vi "(Sub) Write CMD.vi"(7 "State":T1, 8 "error in (no error)":errorcluster caption="에러 입력(에러 없음)", 10 "Write Data":string) -> (0 "error out":errorcluster caption="에러 출력", 1 "Read Byte":i32, 2 "CMD":string, 3 "Write CMD":string)   [LabVIEW 2017]
uses:
  Controls/(Ctrl) State_Write CMD.ctl
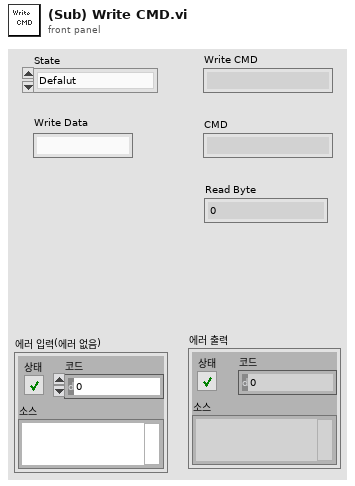
[diagram p1: front panel]
types:
  T1 = typedef "(Ctrl) State_Write CMD.ctl" = enum16{"Defalut", "Set KV", "Set mA", "Get KV", "Get mA", "Get ADC", "HV On", "HV Off", "System State", "HV State", "Opration Mode"}
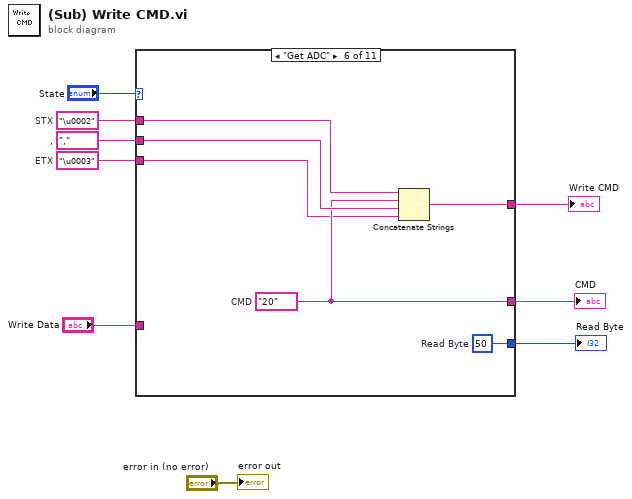
[diagram p0: block diagram]
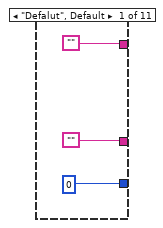
[diagram p2: hidden frame]
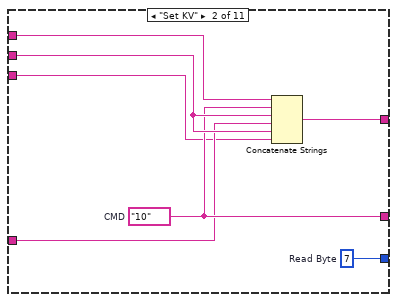
[diagram p3: hidden frame]
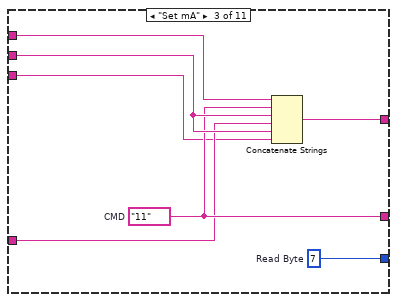
[diagram p4: hidden frame]
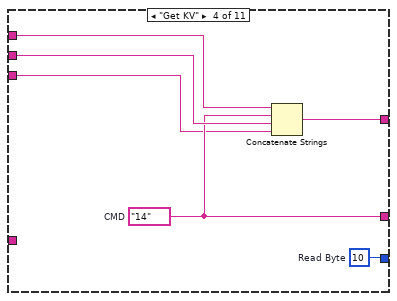
[diagram p5: hidden frame]
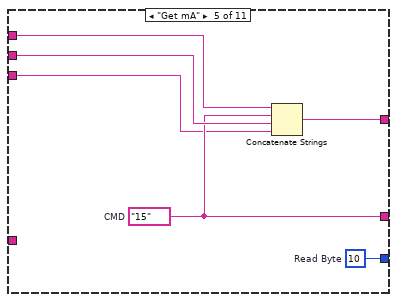
[diagram p6: hidden frame]
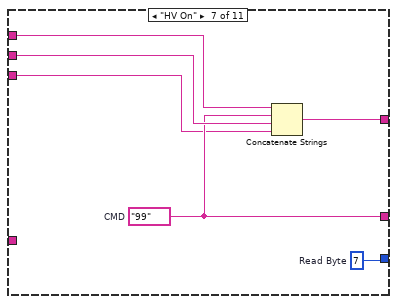
[diagram p7: hidden frame]
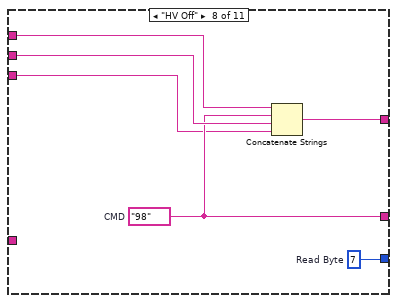
[diagram p8: hidden frame]
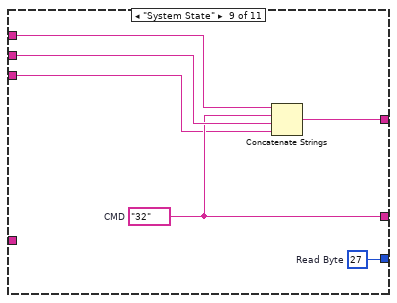
[diagram p9: hidden frame]
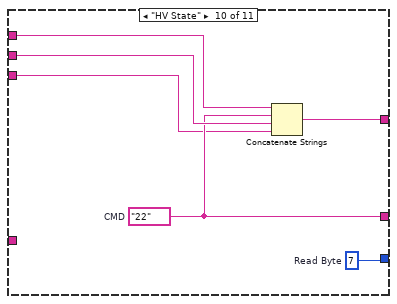
[diagram p10: hidden frame]
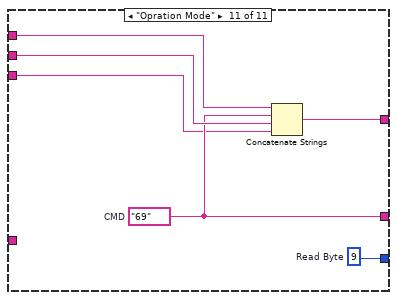
[diagram p11: hidden frame]
diagram:
  w6 = ","  # ,
  w1 = "\u0003"  # ETX
  w7 = "\u0002"  # STX
  n1 = case shown="\"Get ADC\"" "State" {
    tunnel: w7 -> [_ w18 w25 w31 w37 w43 w49 w55 w61 w67 w73]
    tunnel: w6 -> [_ w19 w26 w32 w38 w44 w50 w56 w62 w68 w74]
    tunnel: ["" w17 w24 w30 w36 w42 w48 w54 w60 w66 w72] -> w5
    tunnel: ["" w16 w23 w29 w35 w41 w47 w53 w59 w65 w71] -> w4
    tunnel: "Write Data" -> [_ w15 w22 _ _ _ _ _ _ _ _]
    tunnel: [0 w14 w21 w28 w34 w40 w46 w52 w58 w64 w70] -> w2
    tunnel: w1 -> [_ w13 w20 w27 w33 w39 w45 w51 w57 w63 w69]
    frame "Defalut", Default {
    }
    frame "Set KV" {
      w14 = 7  # Read Byte
      w16 = "10"  # CMD
      n2 = Concatenate Strings(w18, w16, w19, w15, w19, w13) -> (w17:string)
    }
    frame "Set mA" {
      w21 = 7  # Read Byte
      w23 = "11"  # CMD
      n3 = Concatenate Strings(w25, w23, w26, w22, w26, w20) -> (w24:string)
    }
    frame "Get KV" {
      w28 = 10  # Read Byte
      w29 = "14"  # CMD
      n4 = Concatenate Strings(w31, w29, w32, w27) -> (w30:string)
    }
    frame "Get mA" {
      w34 = 10  # Read Byte
      w35 = "15"  # CMD
      n5 = Concatenate Strings(w37, w35, w38, w33) -> (w36:string)
    }
    frame "Get ADC" {
      w40 = 50  # Read Byte
      w41 = "20"  # CMD
      n6 = Concatenate Strings(w43, w41, w44, w39) -> (w42:string)
    }
    frame "HV On" {
      w46 = 7  # Read Byte
      w47 = "99"  # CMD
      n7 = Concatenate Strings(w49, w47, w50, w45) -> (w48:string)
    }
    frame "HV Off" {
      w52 = 7  # Read Byte
      w53 = "98"  # CMD
      n8 = Concatenate Strings(w55, w53, w56, w51) -> (w54:string)
    }
    frame "System State" {
      w58 = 27  # Read Byte
      w59 = "32"  # CMD
      n9 = Concatenate Strings(w61, w59, w62, w57) -> (w60:string)
    }
    frame "HV State" {
      w64 = 7  # Read Byte
      w65 = "22"  # CMD
      n10 = Concatenate Strings(w67, w65, w68, w63) -> (w66:string)
    }
    frame "Opration Mode" {
      w70 = 9  # Read Byte
      w71 = "69"  # CMD
      n11 = Concatenate Strings(w73, w71, w74, w69) -> (w72:string)
    }
  }
  "Write CMD" <- w5
  "CMD" <- w4
  "Read Byte" <- w2
  "error out" <- "error in (no error)"
